vi "SENS_IF_GATE_STAT.vi"(0 "VISA IN":refnum<visa-resource-name>, 1 "IF Gate ON/OFF":bool, 5 "error in":errorcluster, 7 "Channel":i32) -> (14 "VISA Out":refnum<visa-resource-name>, 19 "error out":errorcluster)   [LabVIEW 2018, in "PNA-X.lvlib"]
doc: "SENSe<cnum>:IF:GATE:STATe <boolean> \n(Read-Write) Sets or returns the IF filter gate state. \nParameters \n<cnum> Existing channel number to manipulate. If unspecified, <cnum> is set to 1. \n<boolean> Choose from ON or OFF \nExamples SENS:IF:FILT:GATE:STAT ON \nsense2:if:filter:gate:state 0 \nQuery Syntax SENS:IF:FILTer:SAMPle:COUNt:MODE? \nReturn Type Boolean \nDefault AUTO"
uses:
  PNA-X.lvlib
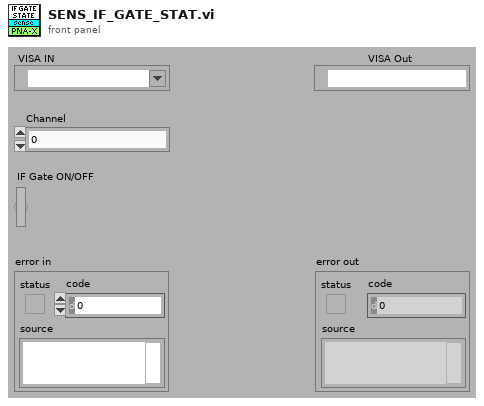
[diagram p1: front panel]
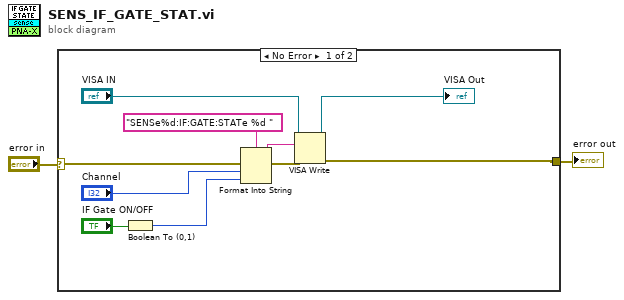
[diagram p0: block diagram]
diagram:
  n1 = case shown="No Error" "error in" {
    selector: "error in" -> [w12 w13]
    tunnel: [w7 w13] -> w1
    frame No Error {
      n2 = Boolean To (0,1)(Boolean="IF Gate ON/OFF") -> (0, 1=w3:i16)
      n3 = Format Into String(format string="SENSe%d:IF:GATE:STATe %d " ("Cmdline"), error in=w12, "Channel", w3) -> (resulting string=w10:string, error out=w11:errorcluster)  [unwired: 1 in]
      n4 = VISA Write(VISA resource name="VISA IN", write buffer=w10, error in (no error)=w11) -> (VISA resource name out=→"VISA Out":refnum<visa-resource-name>, error out=w7:errorcluster)  [unwired: 1 out]
    }
    frame Error {
    }
  }
  "error out" <- w1
